vi "Cleanup.vi"(8 "error in (no error)":errorcluster, 11 "PathTree in":refnum<class "PathTree.lvclass">) -> (0 "error out":errorcluster)   [LabVIEW 2020, in "Advanced Structures.lvlib" / "PathTree.lvclass"]
uses:
  PathTree.lvclass
  PathTreeNode/PathTreeNode.lvclass
  PathTree.lvclass/PathTree.ctl
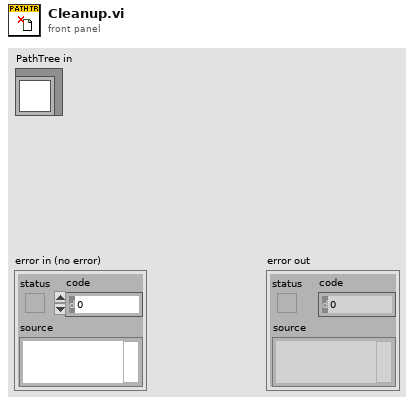
[diagram p1: front panel]
types:
  T1 = typedef "Advanced Structures.lvlib/PathTree.lvclass/Ref Data.ctl" = cluster{"Root":refnum<class>}
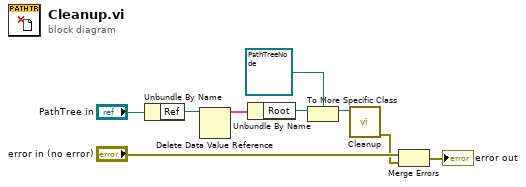
[diagram p0: block diagram]
diagram:
  n1 = Unbundle By Name("PathTree in") -> ("Ref"=w7:refnum<data-value>)
  n2 = Delete Data Value Reference(data value reference=w7) -> (data value=w6:T1)  [unwired: 1 in, 1 out]
  n3 = Unbundle By Name(w6) -> ("Root"=w5:refnum<class>)
  n4 = To More Specific Class(target class=refnum<class "PathTreeNode.lvclass"> refnum ("Advanced Structures.lvlib:PathTreeNode.lvclass"), reference=w5) -> (specific class reference=w4:refnum<class "PathTreeNode.lvclass">)  [unwired: 1 in, 1 out]
  n5 = call "Cleanup.vi"("PathTreeNode in"=w4) -> ("error out"=w1:errorcluster)  [unwired: 10 in]
  n6 = Merge Errors("error in (no error)", w1) -> (→"error out":errorcluster)
